vi "ReadArduino.vi"(9 "Array in":dbl[][](array[numeric]), 10 "String in":string, 11 "VISA Refnum in":refnum<visa-resource-name>) -> (0 "error out":errorcluster, 1 "Array out":dbl[][](array[numeric]), 2 "String out":string, 3 "VISA Refnum out":refnum<visa-resource-name>)   [LabVIEW 2019]
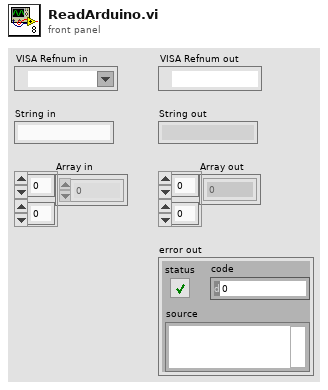
[diagram p1: front panel]
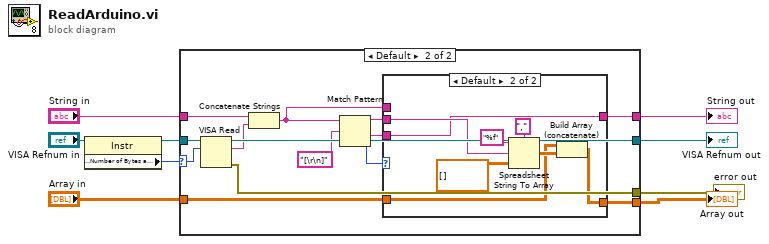
[diagram p0: block diagram]
diagram:
  n1 = property class="Instr"(reference="VISA Refnum in") -> (reference out=w2:refnum<visa-resource-name>, "Serial Settings:Number of Bytes at Serial Port"=w6:u32)  [unwired: 1 in, 1 out]
  n2 = case shown="Default" w6 {
    selector: w6 -> [_ w13]
    tunnel: w2 -> [w12 w26]
    tunnel: [_ w25] -> w3
    tunnel: [w12 w24] -> w4
    tunnel: "String in" -> [w11 w23]
    tunnel: [w11 w16] -> w7
    tunnel: [w10 w19] -> w9
    tunnel: "Array in" -> [w10 w18]
    frame 0 {
    }
    frame Default {
      n3 = VISA Read(VISA resource name=w26, byte count=w13) -> (VISA resource name out=w24:refnum<visa-resource-name>, read buffer=w22:string, error out=w25:errorcluster)  [unwired: 1 in, 1 out]
      n4 = Concatenate Strings(w23, w22) -> (w14:string)
      n5 = Match Pattern(string=w14, regular expression="[\r\n]") -> (before substring=w20:string, after substring=w15:string, offset past match=w17:i32)  [unwired: 1 in, 1 out]
      n6 = case shown="Default" w17 {
        tunnel: w20 -> [_ w33]
        tunnel: [w28 w31] -> w19
        tunnel: w18 -> [w28 w30]
        tunnel: [w27 w29] -> w16
        tunnel: w15 -> [_ w29]
        tunnel: w14 -> [w27 _]
        frame -1 {
        }
        frame Default {
          n7 = Spreadsheet String To Array(delimiter (Tab)=",", format string="%f", spreadsheet string=w33, array type (2D Dbl)=dbl[][] []) -> (array=w32:dbl[][])
          n8 = Build Array (concatenate)(w30, w32) -> (w31:dbl[][])
        }
      }
    }
  }
  "Array out" <- w9
  "String out" <- w7
  "VISA Refnum out" <- w4
  "error out" <- w3
